vi "ToString.vi"(8 "error in (no error)":errorcluster, 11 "Error in":refnum<class "Error.lvclass">) -> (0 "error out":errorcluster, 2 "String":string, 3 "Error out":refnum<class "Error.lvclass">)   [LabVIEW 2017, in "Transparent Assertions.lvlib" / "Constraints.lvlib" / "Error.lvclass"]
doc: "Returns a string representation of the object."
uses:
  Error.lvclass
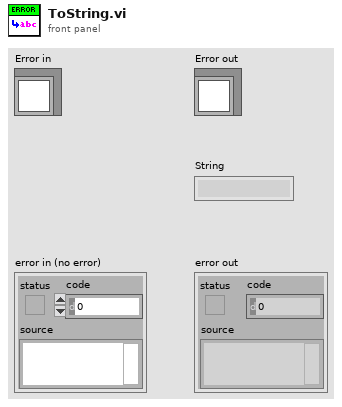
[diagram p1: front panel]
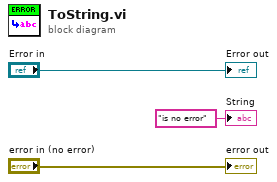
[diagram p0: block diagram]
diagram:
  "error out" <- "error in (no error)"
  "Error out" <- "Error in"
  "String" <- "is no error" ("String")
